vi "Array Of Clusters - Read Age.vi"(8 "error in (no error)":errorcluster, 11 "input array":T1(array[cluster])) -> (0 "error out":errorcluster, 3 "output array":T1(array[cluster]))   [LabVIEW 2012]
uses:
  ClassDefinitions/SimpleClassWithProperties/myClass.lvclass
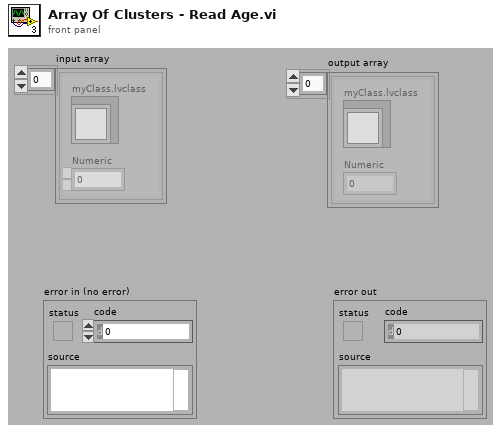
[diagram p1: front panel]
types:
  T1 = cluster{"myClass.lvclass":refnum<class "myClass.lvclass">, "Numeric":dbl}[]
  T2 = cluster{"myClass.lvclass":refnum<class "myClass.lvclass">, "Numeric":dbl}
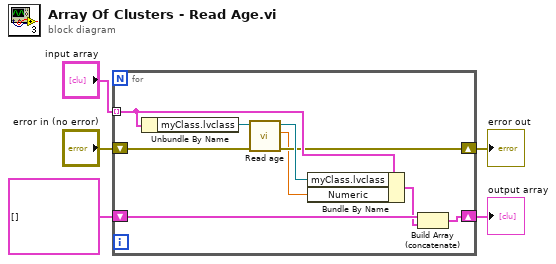
[diagram p0: block diagram]
diagram:
  n1 = for {
    tunnel: "input array" -> [w12] mode=indexing
    shift-right: [w9] -> w3
    shift-left: T1 [] ("input array") -> [w11]
    shift-right: [w7] -> w1
    shift-left: "error in (no error)" -> [w8]
    n2 = Unbundle By Name(w12) -> ("myClass.lvclass"=w14:refnum<class "myClass.lvclass">)
    n3 = call-dynamic "Read age.vi"("error in (no error)"=w8, "myClass in"=w14) -> ("error out"=w7:errorcluster, "age"=w6:dbl, "myClass out"=w13:refnum<class "myClass.lvclass">)  [unwired: 7 in]
    n4 = Bundle By Name(cluster=w12, "myClass.lvclass"=w13, "Numeric"=w6) -> (w10:T2)
    n5 = Build Array (concatenate)(w11, w10) -> (w9:T1)
  }
  "output array" <- w3
  "error out" <- w1
